vi "sysexec2.vi"() -> ()   [LabVIEW 2011]
panel:
  out "standard error":string
  out "standard output":string
  in  "text":string="ls -al /tmp/atlas/ambientpipe "
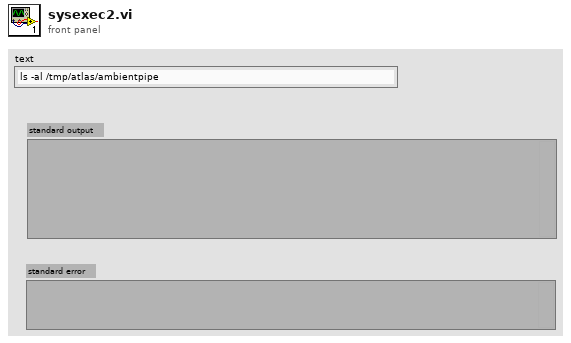
[diagram p1: front panel]
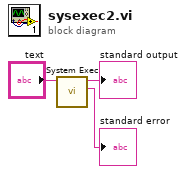
[diagram p0: block diagram]
diagram:
  n1 = call <vilib>:"System Exec.vi"("command line"="text") -> ("standard error"=→"standard error":string, "standard output"=→"standard output":string)  [unwired: 7 in, 2 out]
